vi "灵敏度判定.vi"(0 "曲线引用":refnum<vi>, 1 "灵敏度":T1, 3 "错误输入":errorcluster) -> (7 "曲线引用输出":refnum<vi>, 8 "OK？":bool, 10 "错误输出":errorcluster)   [LabVIEW 2018]
uses:
  Global_Variable/Global.vi
  Global_Variable/A180648.vi
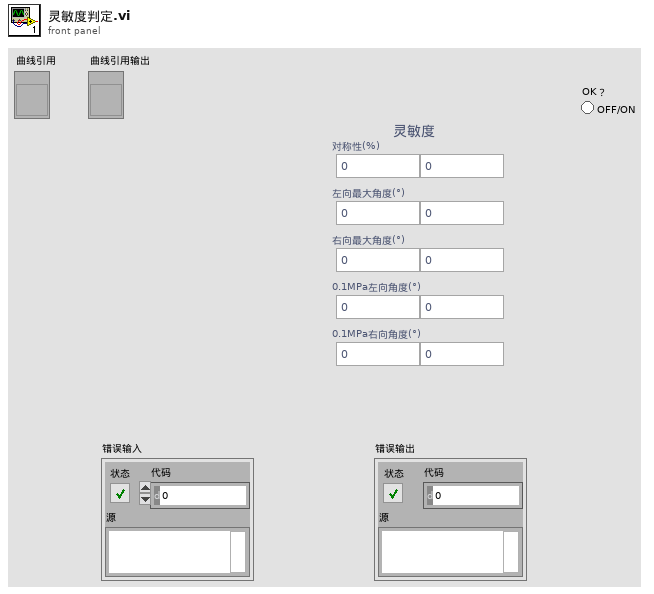
[diagram p1: front panel]
types:
  T1 = cluster{"对称性(%)":cluster{"下限":dbl, "上限":dbl}, "左向最大角度(°)":cluster{"下限":dbl, "上限":dbl}, "右向最大角度(°)":cluster{"下限":dbl, "上限":dbl}, "0.1MPa左向角度(°)":cluster{"下限":dbl, "上限":dbl}, "0.1MPa右向角度(°)":cluster{"下限":dbl, "上限":dbl}}
  T2 = enum32{"空载", "功能", "力特性", "传感器特性", "电流特性", "振动NVH", "逆向空载", "完成"}
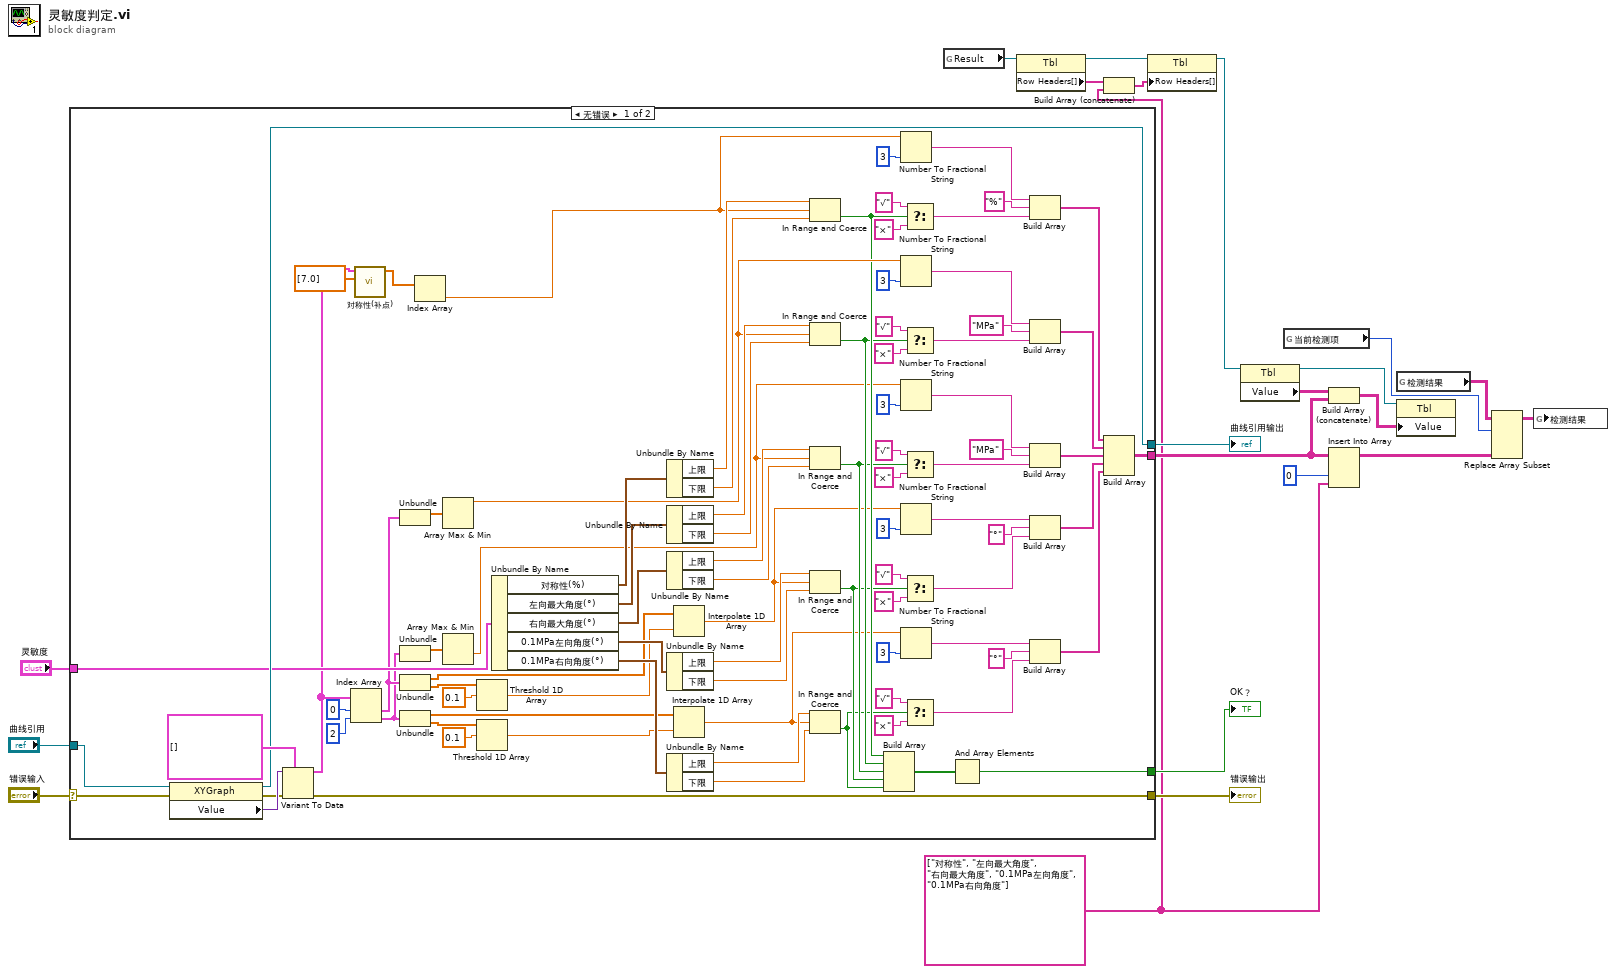
[diagram p0: block diagram]
diagram:
  w3 = string[] ["对称性", "左向最大角度", "右向最大角度", "0.1MPa左向角度", "0.1MPa右向角度"] ("列首字符串[]")
  n1 = case shown="无错误" "错误输入" {
    selector: "错误输入" -> [w107 w111]
    tunnel: [w104 w111] -> w20
    tunnel: "曲线引用" -> [w103 w110]
    tunnel: [w106 w110] -> w18
    tunnel: [w62 _] -> w17
    tunnel: "灵敏度" -> [w102 _]
    tunnel: [w61 _] -> w4
    frame No Error {
      n2 = property class="XYGraph"(reference=w103, error in=w107) -> (reference out=w106:refnum<vi>, error out=w105:errorcluster, "Value"=w109:variant)
      n3 = Variant To Data(error in=w105, type=cluster{dbl[], dbl[]}[] [], Variant=w109) -> (data=w25:cluster{dbl[], dbl[]}[], error out=w104:errorcluster)
      n4 = Index Array(array=w25, index #1=0 ("索引"), index #2=2 ("索引")) -> (element #1=w41:cluster{dbl[], dbl[]}, element #2=w40:cluster{dbl[], dbl[]})
      n5 = call "对称性(补点).vi"("检测点"=dbl[] [7.0], "XY图"=w25) -> ("对称性"=w23:dbl[])  [unwired: 9 in]
      n6 = Unbundle(w41) -> (w83:dbl[])  [unwired: 1 out]
      n7 = Unbundle(w40) -> (w73:dbl[])  [unwired: 1 out]
      n8 = Unbundle(w41) -> (w34:dbl[], w35:dbl[])
      n9 = Unbundle(w40) -> (w29:dbl[], w30:dbl[])
      n10 = Index Array(array=w23) -> (element=w22:dbl)  [unwired: 1 in]
      n11 = Array Max & Min(array=w83) -> (max value=w82:dbl)  [unwired: 3 out]
      n12 = Array Max & Min(array=w73) -> (min value=w60:dbl)  [unwired: 3 out]
      n13 = Threshold 1D Array(2:0.1 ("阈值y"), 3:w35) -> (0:w38:dbl)  [unwired: 1 in]
      n14 = Threshold 1D Array(2:0.1 ("阈值y"), 3:w30) -> (0:w33:dbl)  [unwired: 1 in]
      n15 = Unbundle By Name(w102) -> ("对称性(%)"=w101:cluster{"下限":dbl, "上限":dbl}, "左向最大角度(°)"=w84:cluster{"下限":dbl, "上限":dbl}, "右向最大角度(°)"=w72:cluster{"下限":dbl, "上限":dbl}, "0.1MPa左向角度(°)"=w57:cluster{"下限":dbl, "上限":dbl}, "0.1MPa右向角度(°)"=w42:cluster{"下限":dbl, "上限":dbl})
      n16 = Unbundle By Name(w101) -> ("上限"=w100:dbl, "下限"=w99:dbl)
      n17 = Unbundle By Name(w84) -> ("上限"=w85:dbl, "下限"=w86:dbl)
      n18 = Unbundle By Name(w72) -> ("上限"=w81:dbl, "下限"=w80:dbl)
      n19 = Unbundle By Name(w57) -> ("上限"=w56:dbl, "下限"=w58:dbl)
      n20 = Unbundle By Name(w42) -> ("上限"=w48:dbl, "下限"=w47:dbl)
      n21 = Interpolate 1D Array(1:w38, 2:w34) -> (0:w37:dbl)
      n22 = Interpolate 1D Array(1:w33, 2:w29) -> (0:w31:dbl)
      n23 = In Range and Coerce(upper limit=w100, x=w22, lower limit=w99) -> (In Range?=w68:bool)  [unwired: 1 out]
      n24 = In Range and Coerce(upper limit=w85, x=w82, lower limit=w86) -> (In Range?=w66:bool)  [unwired: 1 out]
      n25 = In Range and Coerce(upper limit=w81, x=w60, lower limit=w80) -> (In Range?=w64:bool)  [unwired: 1 out]
      n26 = In Range and Coerce(upper limit=w56, x=w37, lower limit=w58) -> (In Range?=w52:bool)  [unwired: 1 out]
      n27 = In Range and Coerce(upper limit=w48, x=w31, lower limit=w47) -> (In Range?=w26:bool)  [unwired: 1 out]
      n28 = Build Array(w68, w66, w64, w52, w26) -> (w63:bool[])
      n29 = Number To Fractional String(number=w22, precision (6)=i16 3 ("精度(6)")) -> (F-format string=w97:string)  [unwired: 2 in]
      n30 = Number To Fractional String(number=w82, precision (6)=i16 3 ("精度(6)")) -> (F-format string=w88:string)  [unwired: 2 in]
      n31 = Number To Fractional String(number=w60, precision (6)=i16 3 ("精度(6)")) -> (F-format string=w78:string)  [unwired: 2 in]
      n32 = Number To Fractional String(number=w37, precision (6)=i16 3 ("精度(6)")) -> (F-format string=w55:string)  [unwired: 2 in]
      n33 = Number To Fractional String(number=w31, precision (6)=i16 3 ("精度(6)")) -> (F-format string=w50:string)  [unwired: 2 in]
      n34 = Select(t="√" ("元素"), s=w68, f="×" ("元素")) -> (s? t:f=w93:string)
      n35 = Select(t="√" ("元素"), s=w66, f="×" ("元素")) -> (s? t:f=w92:string)
      n36 = Select(t="√" ("元素"), s=w64, f="×" ("元素")) -> (s? t:f=w74:string)
      n37 = Select(t="√" ("元素"), s=w52, f="×" ("元素")) -> (s? t:f=w45:string)
      n38 = Select(t="√" ("元素"), s=w26, f="×" ("元素")) -> (s? t:f=w43:string)
      n39 = And Array Elements(Boolean array=w63) -> (logical AND=w62:bool)
      n40 = Build Array(w97, "%" ("元素"), w93) -> (w69:string[])
      n41 = Build Array(w88, "MPa" ("元素"), w92) -> (w67:string[])
      n42 = Build Array(w78, "MPa" ("元素"), w74) -> (w65:string[])
      n43 = Build Array(w55, "°" ("元素"), w45) -> (w53:string[])
      n44 = Build Array(w50, "°" ("元素"), w43) -> (w36:string[])
      n45 = Build Array(w69, w67, w65, w53, w36) -> (w61:string[][])
    }
    frame Error {
    }
  }
  "错误输出" <- w20
  "曲线引用输出" <- w18
  "OK？" <- w17
  n46 = global read "Global.vi" "Result"() -> (w13:refnum<vi>)
  n47 = property class="Tbl"(reference=w13) -> (reference out=w12:refnum<vi>, "Row Headers[]"=w10:string[])  [unwired: 1 in, 1 out]
  n48 = Build Array (concatenate)(w10, w3) -> (w9:string[])
  n49 = property class="Tbl"(reference=w12, "Row Headers[]"=w9) -> (reference out=w11:refnum<vi>)  [unwired: 1 in, 1 out]
  n50 = property class="Tbl"(reference=w11) -> (reference out=w16:refnum<vi>, "Value"=w15:string[][])  [unwired: 1 in, 1 out]
  n51 = global read "A180648.vi" "当前检测项"() -> (w6:T2)
  n52 = Build Array (concatenate)(w15, w4) -> (w14:string[][])
  n53 = Insert Into Array(array=w4, index (col)=0 ("禁用的索引 (列)"), new element=w3) -> (w1:string[][])  [unwired: 1 in]
  n54 = global read "A180648.vi" "检测结果"() -> (w7:string[][][])
  n55 = property class="Tbl"(reference=w16, "Value"=w14) -> ()  [unwired: 1 in, 2 out]
  n56 = Replace Array Subset(array=w7, new element=w1, index (dim 0)=w6) -> (w5:string[][][])  [unwired: 2 in]
  n57 = global write "A180648.vi" "检测结果"(w5) -> ()
